vi "Configure Hardware.vi"(8 "error in (no error)":errorcluster, 11 "Hardware Resources in":T1) -> (0 "error out":errorcluster, 3 "Hardware Resources out":T1)   [LabVIEW 2026, in "Acquisition.lvlib"]
doc: "Configure the hardware."
uses:
  Acquisition.lvlib
  Hardware Configuration.ctl
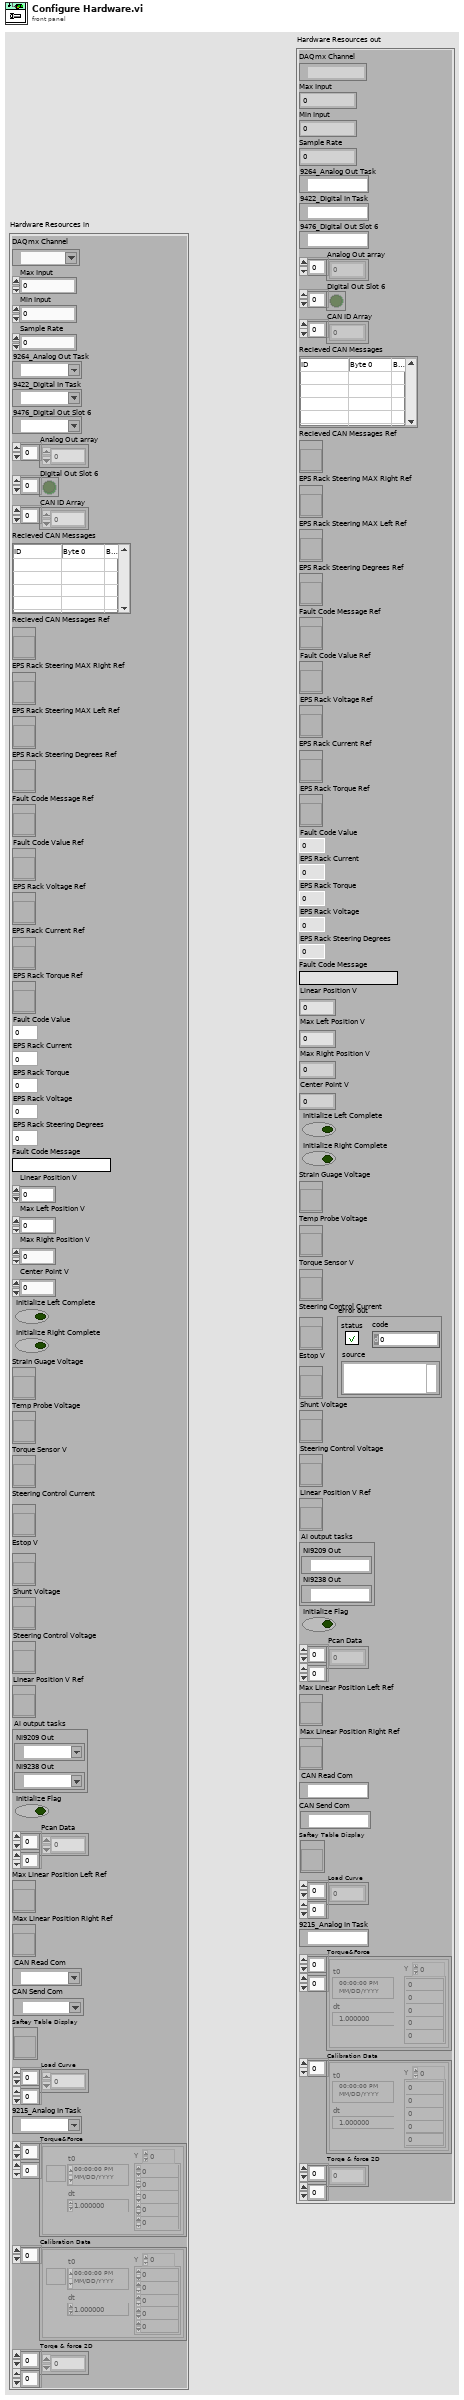
[diagram p1: front panel]
types:
  T1 = typedef "Acquisition.lvlib/Hardware Configuration.ctl" = cluster{"DAQmx Channel":tag, "Max Input":dbl, "Min Input":dbl, "Sample Rate":dbl, "9264_Analog Out Task":refnum<k21>, "9422_Digital In Task":refnum<k21>, "9476_Digital Out Slot 6":refnum<k21>, "Analog Out array":dbl[], "Digital Out Slot 6":bool[], "CAN ID Array":u32[], "Recieved CAN Messages ":string[][], "Recieved CAN Messages Ref":refnum<vi>, "EPS Rack Steering MAX Right Ref":refnum<vi>, "EPS Rack Steering MAX Left Ref":refnum<vi>, "EPS Rack Steering Degrees Ref":refnum<vi>, "Fault Code Message Ref":refnum<vi>, "Fault Code Value Ref":refnum<vi>, "EPS Rack Voltage Ref":refnum<vi>, "EPS Rack Current Ref":refnum<vi>, "EPS Rack Torque Ref":refnum<vi>, "Fault Code Value":dbl, "EPS Rack Current":dbl, "EPS Rack Torque":dbl, "EPS Rack Voltage":dbl, "EPS Rack Steering Degrees":dbl, "Fault Code Message":string, "Linear Position V":dbl, "Max Left Position V":dbl, "Max Right Position V":dbl, "Center Point V":dbl, "Initialize Left Complete":bool, "Initialize Right Complete":bool, "Strain Guage Voltage":refnum<vi>, "Temp Probe Voltage":refnum<vi>, "Torque Sensor V":refnum<vi>, "Steering Control Current":refnum<vi>, "Estop V":refnum<vi>, "Shunt Voltage":refnum<vi>, "Steering Control Voltage":refnum<vi>, "Linear Position V Ref":refnum<vi>, "Ai output tasks":cluster{"NI9209 Out":refnum<k21>, "NI9238 Out":refnum<k21>}, "Initialize Flag":bool, "Pcan Data":dbl[][], "Max Linear Position Left Ref":refnum<vi>, "Max Linear Position Right Ref":refnum<vi>, "CAN Read Com":refnum<k21>, "CAN Send Com":refnum<k21>, "Saftey Table Display":refnum<vi>, "Load Curve":dbl[][], "9215_Analog In Task":refnum<k21>, "Torque&Force":waveform(dbl)[][], "Calibration Data":waveform(dbl)[], "Torqe & force 2D":dbl[][]}
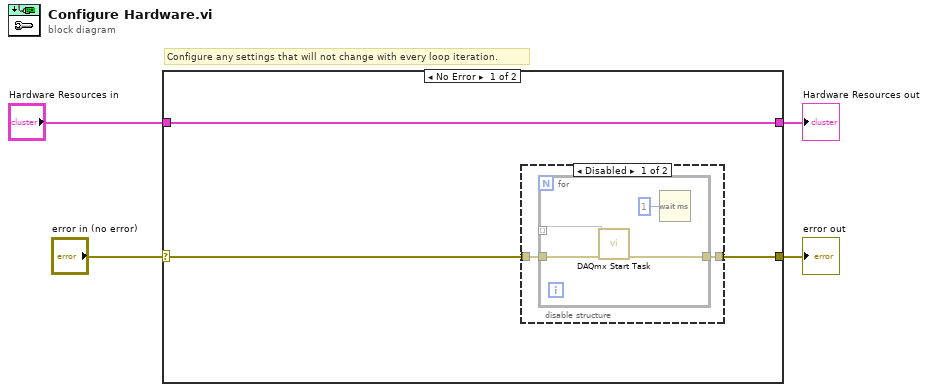
[diagram p0: block diagram]
diagram:
  # "Configure any settings that will not change with every loop iteration."
  n1 = case shown="No Error" "error in (no error)" {
    selector: "error in (no error)" -> [w5 w15]
    tunnel: [w6 w15] -> w3
    tunnel: "Hardware Resources in" -> [w7 w16]
    tunnel: [w7 w16] -> w1
    frame No Error {
      n2 = disable-structure shown="Disabled" {
        disable-tunnel: [w9 w14] -> w6
        disable-tunnel: w5 -> [w8 w14]
        frame Disabled {
          n3 = for {
            tunnel: [w13] -> w9
            tunnel: w8 -> [w12]
            tunnel: _ -> [w11] mode=indexing
            n4 = call <vilib>:"DAQmx Start Task.vi"("task/channels in"=w11, "error in"=w12) -> ("error out"=w13:errorcluster)  [unwired: 12 in, 1 out]
            n5 = Wait (ms)(milliseconds to wait=u32 1) -> ()  [unwired: 1 out]
          }
        }
        frame Enabled {
        }
      }
    }
    frame Error {
    }
  }
  "Hardware Resources out" <- w1
  "error out" <- w3
